vi "Shutdown.vi"(8 "error in (no error)":errorcluster) -> (0 "error out":errorcluster)   [LabVIEW 2014]
uses:
  PacDriveSDK/dlls/PacDrive32.dll
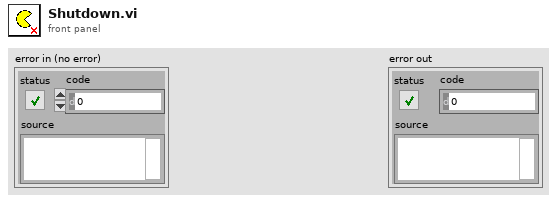
[diagram p1: front panel]
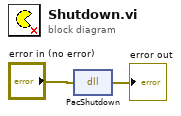
[diagram p0: block diagram]
diagram:
  n1 = dll-call lib="C:/FRC4153/2015/Driverstation/RecycleRush2015DriverStation/LEDdriver/PacDriveSDK/dlls/PacDrive32.dll" fn="PacShutdown"(error in="error in (no error)") -> (error out=→"error out":errorcluster)  [unwired: 3 in, 1 out]
